vi "HEWH Check Element Cutout.vi"(8 "Error In":errorcluster, 9 "Full Cutout":bool, 10 "HEWH Specific DAQ":T1, 11 "Test Conditions":T5 {"Time" format="%<%H:%M:%S>t"}) -> (0 "Error Out":errorcluster, 3 "Go to Draw!":bool)   [LabVIEW 2016]
uses:
  Type Definitions/PRAT Test.ctl
  Utility/Save File/File Setup (Public)/Type Definition/Save File HEWH Heating Control Mode.ctl
  Draw Water Specific/Type Definitions/Terminate Draw Conditions.ctl
  Type Definitions/HEWH Start Conditions.ctl
  Draw Water Specific/Type Definitions/Check Special Condtions.ctl
  Draw Water Specific/Type Definitions/HEWH Special Condition Check.ctl
  Type Definitions/HEWH Draw Flag ENUM.ctl
  Type Definitions/HEWH Specific DAQ.ctl
  Type Definitions/HEWH Power Data.ctl
  Type Definitions/HEWH Power Elements.ctl
  Utility/Type Definitions/UTILITY Power Analyzer.ctl
  Utility/Save File/File Setup.lvlib
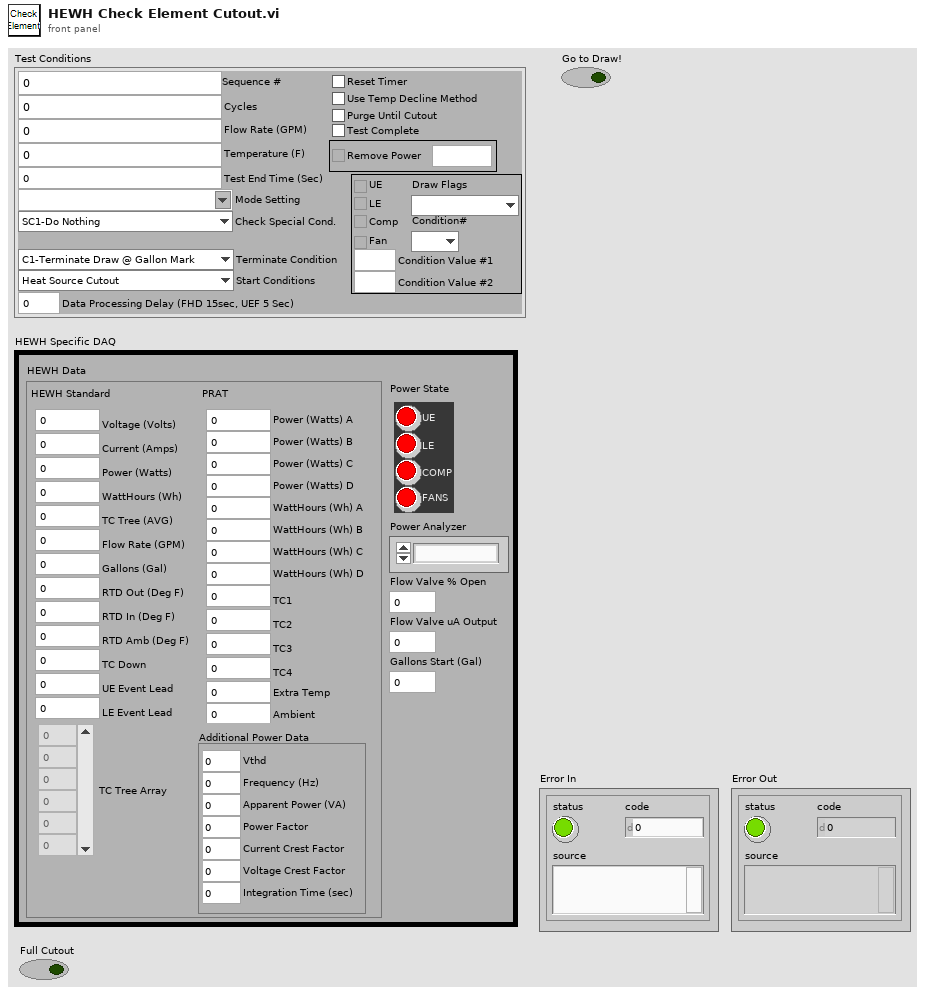
[diagram p1: front panel]
types:
  T1 = typedef "HEWH Specific DAQ.ctl" = cluster{"HEWH Data":T2, "Flow Valve % Open":dbl, "Power State":T3, "Power Analyzer":T4, "Flow Valve uA Output":i32, "Gallons Start (Gal)":dbl}
  T2 = typedef "HEWH Power Data.ctl" = cluster{"HEWH Standard":cluster{"Voltage (Volts)":dbl, "Current (Amps)":dbl, "Power (Watts)":dbl, "WattHours (Wh)":dbl, "TC Tree (AVG)":dbl, "Flow Rate (GPM)":dbl, "Gallons (Gal)":dbl, "RTD Out (Deg F)":dbl, "RTD In (Deg F)":dbl, "RTD Amb (Deg F)":dbl, "TC Down":dbl, "UE Event Lead":i32, "LE Event Lead":i32, "TC Tree Array":dbl[]}, "PRAT":cluster{"Power (Watts) A":dbl, "Power (Watts) B":dbl, "Power (Watts) C":dbl, "Power (Watts) D":dbl, "TC1":dbl, "TC2":dbl, "TC3":dbl, "TC4":dbl, "WattHours (Wh) A":dbl, "WattHours (Wh) B":dbl, "WattHours (Wh) C":dbl, "WattHours (Wh) D":dbl, "Ambient":dbl, "Extra Temp":dbl}, "Additional Power Data":cluster{"Vthd":dbl, "Frequency (Hz)":dbl, "Apparent Power (VA)":dbl, "Power Factor":dbl, "Current Crest Factor":dbl, "Voltage Crest Factor":dbl, "Integration Time (sec)":dbl}}
  T3 = typedef "HEWH Power Elements.ctl" = cluster{"UE":bool, "LE":bool, "COMP":bool, "FANS":bool}
  T4 = typedef "UTILITY Power Analyzer.ctl" = enum16{"", "APLUS", "WT210", "WT500", "WT300", "OSI", "Debug", "WT230", "WT300_1", "WT300_2"}
  T5 = typedef "PRAT Test.ctl" = cluster{"Sequence #":dbl, "Cycles":i32, "Mode Setting":T6, "Flow Rate (GPM)":dbl, "Temperature (F)":dbl, "Reset Timer":bool, "Use Temp Decline Method":bool, "Terminate Condition":T7, "Condition Value #1":dbl, "UE":bool, "LE":bool, "Comp":bool, "Fan":bool, "Test End Time (Sec)":dbl, "Purge Until Cutout":bool, "Start Conditions":T8, "Condition Value #2":dbl, "Remove Power":bool, "Time":dbl, "Check Special Cond.":T9, "Condition#":T10, "Draw Flags":T11, "Data Processing Delay (FHD 15sec, UEF 5 Sec)":dbl, "Test Complete":bool}
  T6 = typedef "File Setup.lvlib/Save File HEWH Heating Control Mode.ctl" = string
  T7 = typedef "Terminate Draw Conditions.ctl" = enum16{"C1-Terminate Draw @ Gallon Mark", "C2-Special Last Draw (HU Test)", "C3-RTD Out <=", "C4-Mean Tank Temp <=", "C5-Decrease RTD Out (Deg F)", "C6-Time (Seconds)", "C7-Until Any Heat Source", "C8-Specific Heat Source", "C9-Do Nothing"}
  T8 = typedef "HEWH Start Conditions.ctl" = enum16{"Heat Source Cutout", "At Time (Seconds)", "Every X (Seconds)", "T2 >= X° Below Setpoint", "Seconds From Complete", "Wait for LE & Comp Cutout", "Wait for Comp Cutout", "Wait for LE Cutout", "Wait for UE Cutout"}
  T9 = typedef "Check Special Condtions.ctl" = enum16{"SC1-Do Nothing", "SC2-Check Heat Source (On-C2/Off-C1)", "SC3-Check Skip Condition", "SC4-Check Heat Source ON/Fail"}
  T10 = typedef "HEWH Special Condition Check.ctl" = enum16{"N/A", "C1", "C2", "Reset/Fail", "Skip Draw Sequence"}
  T11 = typedef "HEWH Draw Flag ENUM.ctl" = enum16{"N/A", "None(0)", "Sml(1)", "Med(2)", "SmlMed(3)", "Lrg(4)", "SmlLrg(5)", "MedLrg(6)", "SmlMedLrg(7)"}
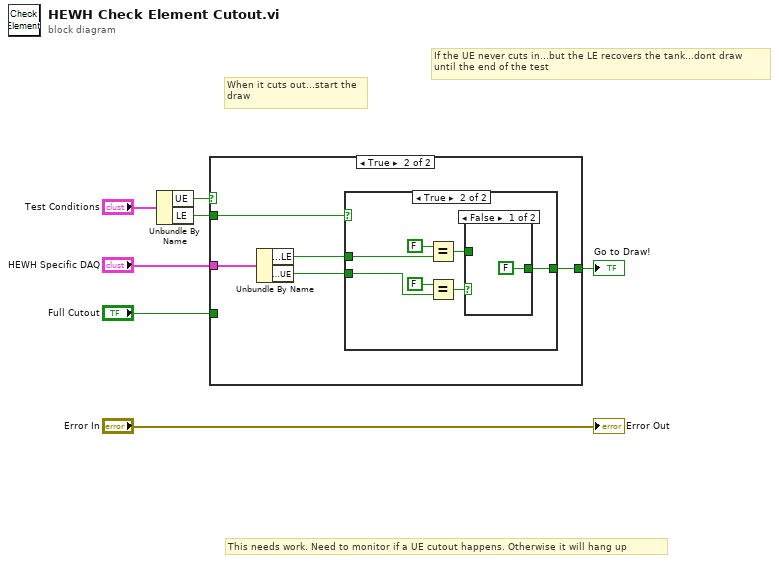
[diagram p0: block diagram]
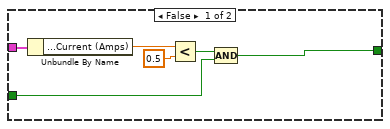
[diagram p2: hidden frame]
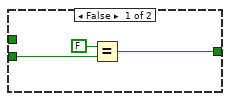
[diagram p3: hidden frame]
diagram:
  # "This needs work. Need to monitor if a UE cutout happens. Otherwise it will hang up"
  # "If the UE never cuts in...but the LE recovers the tank...dont draw \nuntil the end of the test"
  # "When it cuts out...start the\ndraw"
  n1 = Unbundle By Name("Test Conditions") -> ("UE"=w4:bool, "LE"=w7:bool)
  n2 = case shown="True" w4 {
    tunnel: [w8 w15] -> w6
    tunnel: "HEWH Specific DAQ" -> [w12 w18]
    tunnel: "Full Cutout" -> [w9 _]
    tunnel: w7 -> [_ w17]
    frame False {
      n3 = Unbundle By Name(w12) -> ("HEWH Data.HEWH Standard.Current (Amps)"=w11:dbl)
      n4 = Less?(x=w11, y=0.5) -> (x < y?=w10:bool)
      n5 = Compound Arithmetic op=AND(w10, w9) -> (w8:bool)
    }
    frame True {
      n6 = Unbundle By Name(w18) -> ("Power State.LE"=w14:bool, "Power State.UE"=w16:bool)
      n7 = case shown="True" w17 {
        tunnel: w16 -> [w20 w27]
        tunnel: [w19 w22] -> w15
        tunnel: w14 -> [_ w25]
        frame False {
          n8 = Equal?(x=FALSE, y=w20) -> (x = y?=w19:bool)
        }
        frame True {
          n9 = Equal?(x=FALSE, y=w25) -> (x = y?=w23:bool)
          n10 = Equal?(x=FALSE, y=w27) -> (x = y?=w24:bool)
          n11 = case shown="False" w24 {
            tunnel: w23 -> [_ w30]
            tunnel: [FALSE ("x") w30] -> w22
            frame False {
            }
            frame True {
            }
          }
        }
      }
    }
  }
  "Go to Draw!" <- w6
  "Error Out" <- "Error In"
